vi "DSF.Memory.BufferPool.Set Buffers.vi"(8 "error in (no error)":errorcluster, 10 "Buffers":refnum<class "DSF.Memory.Buffer.lvclass">[](array[class]), 11 "BufferPool in":refnum<class "DSF.Memory.BufferPool.lvclass">) -> (0 "error out":errorcluster, 3 "BufferPool out":refnum<class "DSF.Memory.BufferPool.lvclass">)   [LabVIEW 2016, in "DSF.Engine.lvlib" / "DSF.Memory.BufferPool.lvclass"]
uses:
  DSF.Memory.BufferPool.lvclass
  Memory.Buffer/DSF.Memory.Buffer.lvclass
  DSF.Memory.BufferPool.lvclass/DSF.Memory.BufferPool.ctl
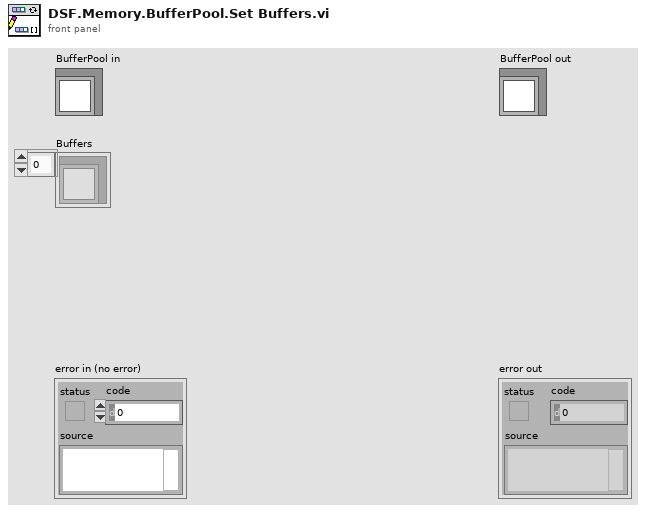
[diagram p1: front panel]
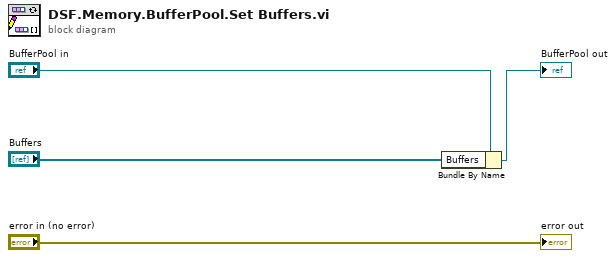
[diagram p0: block diagram]
diagram:
  n1 = Bundle By Name(cluster="BufferPool in", "Buffers"="Buffers") -> (→"BufferPool out":refnum<class "DSF.Memory.BufferPool.lvclass">)
  "error out" <- "error in (no error)"
